vi "aft_xmpl_Delay (PtbyPt).vi"(1 "Delay":i32, 2 "QAM signal":cdb) -> (0 "shifted x":cdb)   [LabVIEW 2019]
uses:
  <vilib>/ptbypt/NI_PtbyPt.lvlib
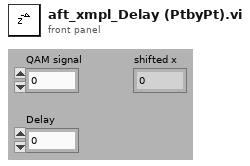
[diagram p1: front panel]
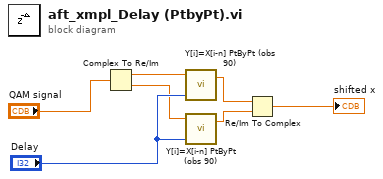
[diagram p0: block diagram]
diagram:
  n1 = Complex To Re/Im(x + iy="QAM signal") -> (x=w6:dbl, y=w4:dbl)
  n2 = call <vilib>:"Y[i]=X[i-n] PtByPt (obs 90).vi"("shifts: n"="Delay", "x"=w6) -> ("shifted x"=w3:dbl)  [unwired: 2 in, 1 out]
  n3 = call <vilib>:"Y[i]=X[i-n] PtByPt (obs 90).vi"("shifts: n"="Delay", "x"=w4) -> ("shifted x"=w2:dbl)  [unwired: 2 in, 1 out]
  n4 = Re/Im To Complex(1:w2, 2:w3) -> (0:→"shifted x":cdb)
